vi "Set #Frames.vi"(8 "error in (no error)":errorcluster, 11 "CCDCamera in":refnum<class "iKon-L.lvclass">) -> (0 "error out":errorcluster, 3 "CCDCamera out":refnum<class "iKon-L.lvclass">)   [LabVIEW 2018, in "iKon-L.lvclass"]
doc: "Set the number of frames in a kinetic series"
uses:
  iKon-L.lvclass
  C:/Users/Denis/Desktop/S4ACS/S4ACS/Sim_CCD/Sim_CCD.lvclass
  Sim_CCD/Sim_CCD.lvclass
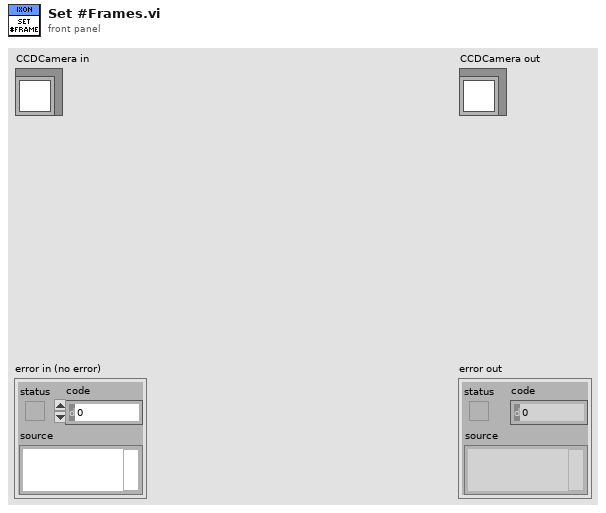
[diagram p1: front panel]
types:
  T1 = cluster{"EXPTIME":dbl, "#FRAMES":u32, "COOLER_POWER_STATUS":u16, "TEMP":i32}
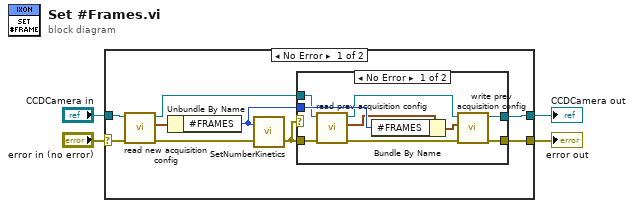
[diagram p0: block diagram]
diagram:
  n1 = case shown="No Error" "error in (no error)" {
    selector: "error in (no error)" -> [w8 w25]
    tunnel: "CCDCamera in" -> [w7 w26]
    tunnel: [w13 w25] -> w2
    tunnel: [w10 w26] -> w1
    frame No Error {
      n2 = call "read new acquisition config.vi"("error in (no error)"=w8, "Simulated_CCD_Camera in"=w7) -> ("error out"=w5:errorcluster, "new acquisition configuration"=w6:T1, "Simulated_CCD_Camera out"=w9:refnum<class "iKon-L.lvclass">)  [unwired: 7 in]
      n3 = Unbundle By Name(w6) -> ("#FRAMES"=w12:u32)
      n4 = call <userlib>:"SetNumberKinetics.vi"("error in (no error)"=w5, "number"=w12) -> ("error out"=w11:errorcluster)  [unwired: 1 out]
      n5 = case shown="No Error" w11 {
        tunnel: [w17 w24] -> w13
        tunnel: w11 -> [w14 w24]
        tunnel: w12 -> [w22 _]
        tunnel: [w16 w23] -> w10
        tunnel: w9 -> [w15 w23]
        frame No Error {
          n6 = call "read prev acquisition config.vi"("error in (no error)"=w14, "Simulated_CCD_Camera in"=w15) -> ("error out"=w18:errorcluster, "prev acquisition configuration"=w21:T1, "Simulated_CCD_Camera out"=w19:refnum<class "iKon-L.lvclass">)  [unwired: 7 in]
          n7 = Bundle By Name(cluster=w21, "#FRAMES"=w22) -> (w20:T1)
          n8 = call "write prev acquisition config.vi"("error in (no error)"=w18, "prev acquisition configuration"=w20, "Simulated_CCD_Camera in"=w19) -> ("error out"=w17:errorcluster, "Simulated_CCD_Camera out"=w16:refnum<class "iKon-L.lvclass">)  [unwired: 7 in]
        }
        frame Error {
        }
      }
    }
    frame Error {
    }
  }
  "error out" <- w2
  "CCDCamera out" <- w1
